vi "Gear_Placer_OperatorAssist.vi"(0 "Start?":bool, 1 "Reset?":bool, 2 "Gear_Peg_Detected?":bool, 3 "Rail_Finished?":bool, 4 "Gate_Finished?":bool, 5 "Gear_Pusher_Finished?":bool, 7 "Place_Gear?":bool) -> (14 "Rail_Track?":bool, 15 "Rail_Reset?":bool, 16 "Gear_Gate_Pos":enum16{"Catch", "Clamp", "Open"}(ring), 17 "Gear_Pusher_Pos":T1)   [LabVIEW 2016]
uses:
  <vilib>/Rock Robotics/WPI/Solenoid/WPI_SolenoidValue.ctl
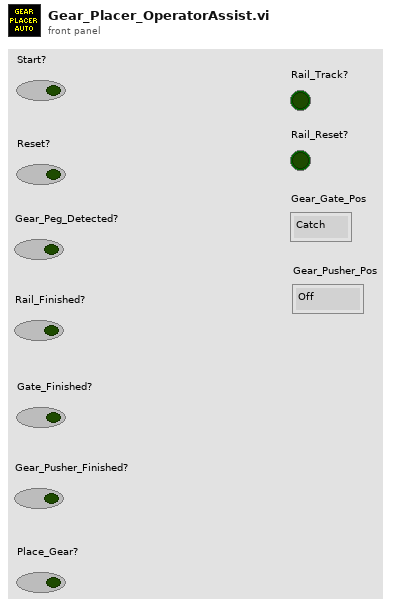
[diagram p1: front panel]
types:
  T1 = typedef "WPI_SolenoidValue.ctl" = enum16{"Off", "On", "Forward", "Reverse"}
  T2 = enum16{"Idle", "Wait for Peg", "Allign To Lift", "Return To Wait", "Arm Gear", "Place Gear", "Return to Ready", "Disarm Gear"}
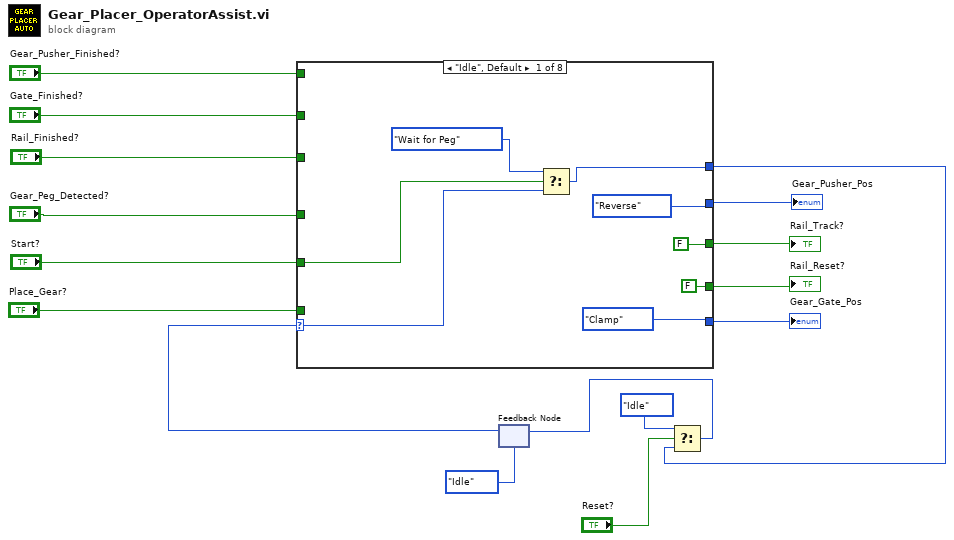
[diagram p0: block diagram]
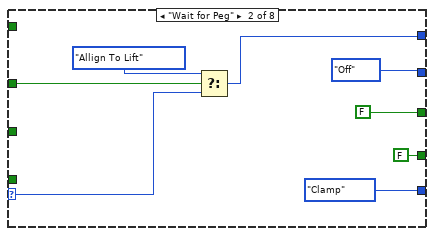
[diagram p2: hidden frame]
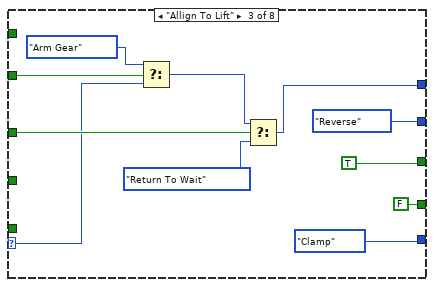
[diagram p3: hidden frame]
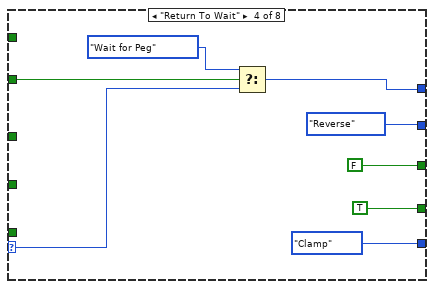
[diagram p4: hidden frame]
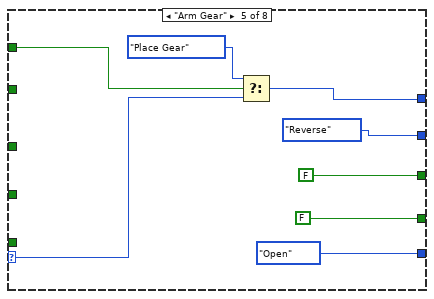
[diagram p5: hidden frame]
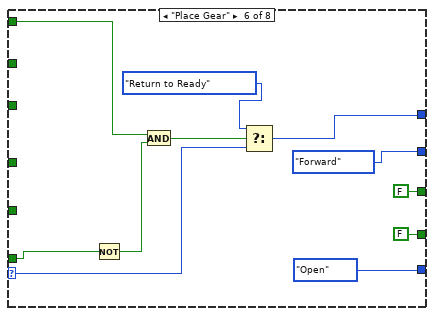
[diagram p6: hidden frame]
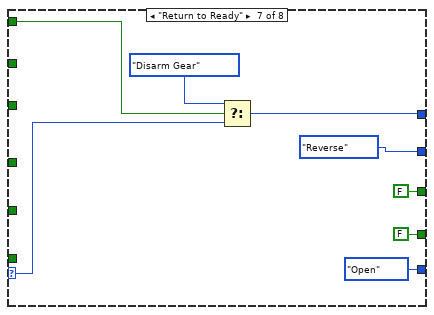
[diagram p7: hidden frame]
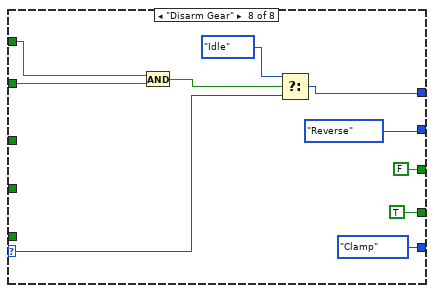
[diagram p8: hidden frame]
diagram:
  n1 = feedback #1(T2."Idle") -> (w7:T2)
  n2 = case shown="\"Idle\", Default" w7 {
    selector: w7 -> [w17 w25 w35 w44 w52 w62 w71 w79]
    tunnel: "Gear_Peg_Detected?" -> [_ w32 w43 _ _ _ _ _]
    tunnel: [w24 w30 w42 w49 w57 w67 w76 w84] -> w5
    tunnel: "Rail_Finished?" -> [_ _ w41 w51 _ _ _ w87]
    tunnel: "Gate_Finished?" -> [_ _ _ _ w59 _ _ w88]
    tunnel: "Start?" -> [w23 _ _ _ _ _ _ _]
    tunnel: "Gear_Pusher_Finished?" -> [_ _ _ _ _ w70 w78 _]
    tunnel: [FALSE FALSE TRUE FALSE FALSE FALSE FALSE FALSE] -> w6
    tunnel: [enum16{"Catch", "Clamp", "Open"}."Clamp" enum16{"Catch", "Clamp", "Open"}."Clamp" enum16{"Catch", "Clamp", "Open"}."Clamp" enum16{"Catch", "Clamp", "Open"}."Clamp" enum16{"Catch", "Clamp", "Open"}."Open" enum16{"Catch", "Clamp", "Open"}."Open" enum16{"Catch", "Clamp", "Open"}."Open" enum16{"Catch", "Clamp", "Open"}."Clamp"] -> w4
    tunnel: [FALSE FALSE FALSE TRUE FALSE FALSE FALSE TRUE] -> w3
    tunnel: [WPI_SolenoidValue."Reverse" ("Value") WPI_SolenoidValue."Off" ("Value") WPI_SolenoidValue."Reverse" ("Value") WPI_SolenoidValue."Reverse" ("Value") WPI_SolenoidValue."Reverse" ("Value") WPI_SolenoidValue."Forward" ("Value") WPI_SolenoidValue."Reverse" ("Value") WPI_SolenoidValue."Reverse" ("Value")] -> w2
    tunnel: "Place_Gear?" -> [_ _ _ _ _ w60 _ _]
    frame "Idle", Default {
      n3 = Select(t=T2."Wait for Peg", s=w23, f=w17) -> (s? t:f=w24:T2)
    }
    frame "Wait for Peg" {
      n4 = Select(t=T2."Allign To Lift", s=w32, f=w25) -> (s? t:f=w30:T2)
    }
    frame "Allign To Lift" {
      n5 = Select(t=T2."Arm Gear", s=w41, f=w35) -> (s? t:f=w33:T2)
      n6 = Select(t=w33, s=w43, f=T2."Return To Wait") -> (s? t:f=w42:T2)
    }
    frame "Return To Wait" {
      n7 = Select(t=T2."Wait for Peg", s=w51, f=w44) -> (s? t:f=w49:T2)
    }
    frame "Arm Gear" {
      n8 = Select(t=T2."Place Gear", s=w59, f=w52) -> (s? t:f=w57:T2)
    }
    frame "Place Gear" {
      n9 = Not(x=w60) -> (.not. x?=w61:bool)
      n10 = And(x=w70, y=w61) -> (x .and. y?=w69:bool)
      n11 = Select(t=T2."Return to Ready", s=w69, f=w62) -> (s? t:f=w67:T2)
    }
    frame "Return to Ready" {
      n12 = Select(t=T2."Disarm Gear", s=w78, f=w71) -> (s? t:f=w76:T2)
    }
    frame "Disarm Gear" {
      n13 = And(x=w88, y=w87) -> (x .and. y?=w86:bool)
      n14 = Select(t=T2."Idle", s=w86, f=w79) -> (s? t:f=w84:T2)
    }
  }
  "Rail_Track?" <- w6
  "Gear_Gate_Pos" <- w4
  "Rail_Reset?" <- w3
  "Gear_Pusher_Pos" <- w2
  n15 = Select(t=T2."Idle", s="Reset?", f=w5) -> (s? t:f=w12:T2)
  n16 = feedback-in #1(w12) -> ()
